vi "MGI RWA Handle Tag or Refnum.vi"(4 "Read State In":T2={"StrToSpecifiedText"=variant, "Specified Data"=variant, "Float Fmt"="%#_13g", "Major Vers"=0, "Options"={"TS Fmt"="", "Int Fmt"="", "Delimiter"=","}}, 6 "Conversion":T1, 8 "Error In":errorcluster, 9 "Anything":variant, 10 "Read String":string) -> (0 "Error Out":errorcluster, 1 "String":string)   [LabVIEW 2020]
doc: "Handle a Tag or Reference datatype, converting to a string or from a string.\n\nAuthored by Shawn D. Walpole\nsupport@mooregoodideas.com\nwww.mooregoodideas.com\n\nCopyright (c) 2010, Moore Good Ideas, Inc.\n\nAll rights reserved.\n\nRedistribution and use in source and binary forms, with or without modification, are permitted provided that the following conditions are met:\n\n * Redistributions of source code must retain the above copyright notice, this list of conditions and the following disclaimer.\n * Redistributions in binary form must reproduce the above copyright notice, this list of conditions and the following disclaimer in the documentation and/or other materials provided with the distribution.\n * Neither the name of Moore Good Ideas, Inc. nor the names of its contributors may be used to endorse or promote products derived from this software without specific prior written permission.\n\nTHIS SOFTWARE IS PROVIDED BY THE COPYRIGHT HOLDERS AND CONTRIBUTORS \"AS IS\" AND ANY EXPRESS OR IMPLIED WARRANTIES, INCLUDING, BUT NOT LIMITED TO, THE IMPLIED WARRANTIES OF MERCHANTABILITY AND FITNESS FOR A PARTICULAR PURPOSE ARE DISCLAIMED. IN NO EVENT SHALL THE COPYRIGHT OWNER OR CONTRIBUTORS BE LIABLE FOR ANY DIRECT, INDIRECT, INCIDENTAL, SPECIAL, EXEMPLARY, OR CONSEQUENTIAL DAMAGES (INCLUDING, BUT NOT LIMITED TO, PROCUREMENT OF SUBSTITUTE GOODS OR SERVICES; LOSS OF USE, DATA, OR PROFITS; OR BUSINESS INTERRUPTION) HOWEVER CAUSED AND ON ANY THEORY OF LIABILITY, WHETHER IN CONTRACT, STRICT LIABILITY, OR TORT (INCLUDING NEGLIGENCE OR OTHERWISE) ARISING IN ANY WAY OUT OF THE USE OF THIS SOFTWARE, EVEN IF ADVISED OF THE POSSIBILITY OF SUCH DAMAGE."
uses:
  <userlib>/_MGI/Read Write Anything/MGI RWA Options Cluster.ctl
  <userlib>/_MGI/Read Write Anything/MGI RWA Tag Lookup Cluster.ctl
  <userlib>/_MGI/Read Write Anything/MGI RWA Convertion Direction Enum.ctl
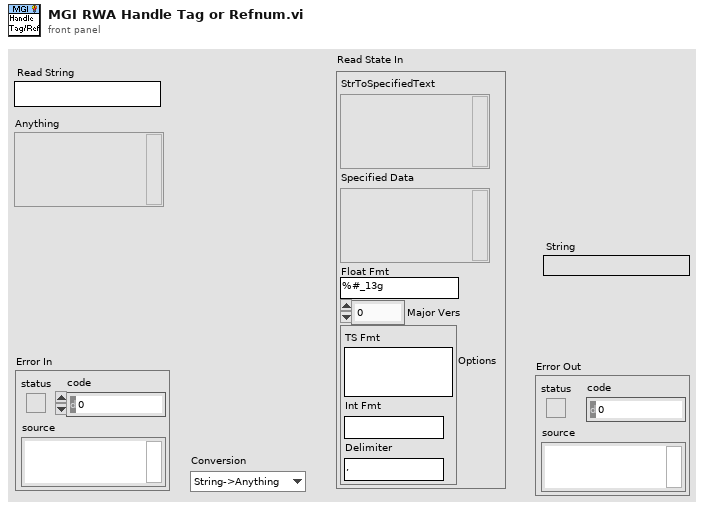
[diagram p1: front panel]
types:
  T1 = typedef "MGI RWA Convertion Direction Enum.ctl" = enum16{"String->Anything", "Anything->String"}
  T2 = typedef "MGI RWA Tag Lookup Cluster.ctl" = cluster{"StrToSpecifiedText":variant, "Specified Data":variant, "Float Fmt":string, "Major Vers":i32, "Options":T3}
  T3 = typedef "MGI RWA Options Cluster.ctl" = cluster{"TS Fmt":string, "Int Fmt":string, "Delimiter":string}
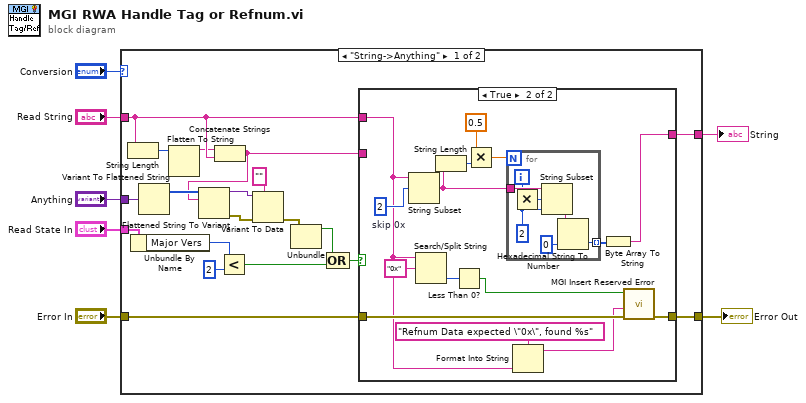
[diagram p0: block diagram]
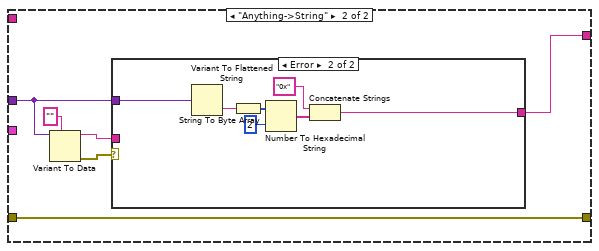
[diagram p3: hidden frame]
diagram:
  n1 = case shown="\"String->Anything\"" "Conversion" {
    tunnel: "Read State In" -> [w22 _]
    tunnel: "Anything" -> [w12 w51]
    tunnel: "Read String" -> [w21 _]
    tunnel: "Error In" -> [w17 w52]
    tunnel: [w16 w52] -> w3
    tunnel: [w15 w53] -> w2
    frame "String->Anything" {
      n2 = String Length(string=w21) -> (length=w20:i32)
      n3 = Unbundle By Name(w22) -> ("Major Vers"=w26:i32)
      n4 = Variant To Flattened String(Variant=w12) -> (1:w11:i16[])  [unwired: 1 out]
      n5 = Flatten To String(anything=w20) -> (data string=w19:string)  [unwired: 3 in, 2 out]
      n6 = Concatenate Strings(w19, w21) -> (w9:string)
      n7 = Flattened String To Variant(6:w9, 7:w11) -> (0:w10:errorcluster, 3:w8:variant)  [unwired: 1 in]
      n8 = Less?(x=w26, y=2) -> (x < y?=w24:bool)
      n9 = Variant To Data(error in=w10, type="", Variant=w8) -> (error out=w13:errorcluster)  [unwired: 1 out]
      n10 = Unbundle(w13) -> ("status"=w23:bool)  [unwired: 2 out]
      n11 = Compound Arithmetic op=OR(w23, w24) -> (w18:bool)
      n12 = case shown="True" w18 {
        tunnel: w21 -> [_ w31]
        tunnel: w17 -> [w27 w33]
        tunnel: [w27 w32] -> w16
        tunnel: [w28 w37] -> w15
        tunnel: w9 -> [w28 _]
        frame False {
        }
        frame True {
          w43 = 2  # skip 0x
          n13 = String Subset(string=w31, offset (0)=w43) -> (substring=w38:string)  [unwired: 1 in]
          n14 = Search/Split String(string=w31, search string/char (-)="0x") -> (offset of match=w35:i32)  [unwired: 1 in, 2 out]
          n15 = String Length(string=w38) -> (length=w41:i32)
          n16 = Less Than 0?(x=w35) -> (x < 0?=w34:bool)
          n17 = Multiply(x=0.5, y=w41) -> (x*y=w39:dbl)
          n18 = for {
            N: w39 -> [_]
            tunnel: w38 -> [w47]
            tunnel: [w49] -> w42 mode=indexing
            i -> [w46]
            w45 = 2 ("length (rest)")
            n19 = Multiply(x=w46, y=w45) -> (x*y=w44:i32)
            n20 = String Subset(string=w47, offset (0)=w44, length (rest)=w45) -> (substring=w48:string)
            n21 = Hexadecimal String To Number(string=w48, default (0uL)=u8 0 ("default (0 U32)")) -> (number=w49:u8)  [unwired: 1 in, 1 out]
          }
          n22 = Format Into String(format string="Refnum Data expected \"0x\", found %s" ("Error Description"), w31) -> (resulting string=w29:string)  [unwired: 2 in, 1 out]
          n23 = Byte Array To String(unsigned byte array=w42) -> (string=w37:string)
          n24 = call <userlib>:"MGI Insert Reserved Error.vi"("Error In"=w33, "Error Description"=w29, "Error? (T)"=w34) -> ("Error Out"=w32:errorcluster)  [unwired: 8 in]
        }
      }
    }
    frame "Anything->String" {
      n25 = Variant To Data(type="", Variant=w51) -> (data=w54:string, error out=w55:errorcluster)  [unwired: 1 in]
      n26 = case shown="Error" w55 {
        tunnel: w54 -> [w57 _]
        tunnel: [w57 w58] -> w53
        tunnel: w51 -> [_ w59]
        frame No Error {
        }
        frame Error {
          n27 = Variant To Flattened String(Variant=w59) -> (data string=w60:string)  [unwired: 1 out]
          n28 = String To Byte Array(string=w60) -> (unsigned byte array=w64:u8[])
          n29 = Number To Hexadecimal String(1:i16 2 ("width (-)"), 2:w64) -> (0:w63:string[])
          n30 = Concatenate Strings("0x", w63) -> (w58:string)
        }
      }
    }
  }
  "Error Out" <- w3
  "String" <- w2
